vi "Engine Config Cluster to DSF Config File.vi"(8 "error in (no error)":errorcluster, 10 "dsf configuration file path":path, 11 "framework configuration":T1) -> (0 "error out":errorcluster)   [LabVIEW 2017, in "DSF Core.lvlib" / "Configuration Session.lvclass"]
uses:
  Configuration/Configuration Session.lvclass
  Configuration/Public/Controls/DSF Engine Framework Configuration.ctl
  Configuration/Public/Controls/DSF Engine Plugin Configuration.ctl
  Configuration/Public/Controls/DSF Timing Info.ctl
  Configuration/Public/Controls/DSF Engine Transfer Group Configuration.ctl
  Configuration/Public/Controls/DSF Direction.ctl
  Configuration/Public/Controls/DSF Engine Transfer Configuration.ctl
  Configuration/Public/Controls/DSF Byte Order.ctl
  Configuration/Public/Controls/DSF Engine Channel Configuration.ctl
  Configuration/Public/Controls/DSF Data Type.ctl
  Configuration/Public/Controls/DSF Settings Info.ctl
  Configuration/Public/Controls/DSF Plugin Info.ctl
  Configuration/Public/Controls/DSF Group Info.ctl
  Configuration/Public/Controls/DSF Transfer Info.ctl
  Configuration/Public/Controls/DSF Channel Info.ctl
  Configuration/Public/Write Item/Write Channel.vi
  Configuration/Public/Write Item/Write Transfer.vi
  Configuration/Public/Write Item/Write Group.vi
  Configuration/Public/Write Item/Write Plugin.vi
  DSF Core.lvlib
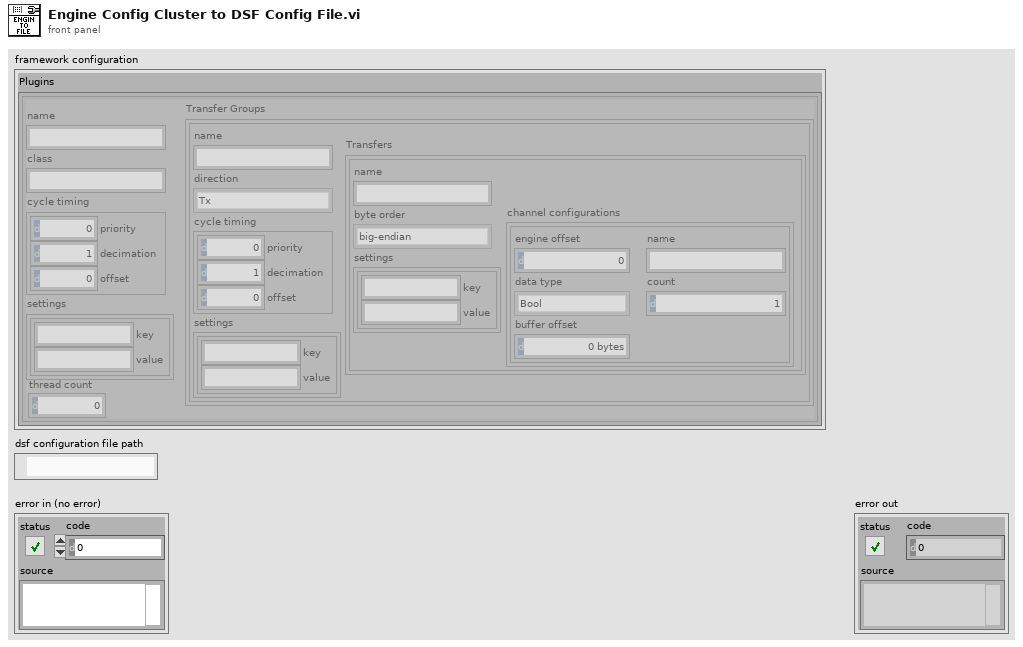
[diagram p1: front panel]
types:
  T1 = typedef "DSF Core.lvlib/DSF Engine Framework Configuration.ctl" = cluster{"Plugins":T2[]}
  T2 = typedef "DSF Core.lvlib/DSF Engine Plugin Configuration.ctl" = cluster{"name":string, "class":string, "cycle timing":T3, "Transfer Groups":T4[], "settings":T10, "thread count":i32}
  T3 = typedef "DSF Core.lvlib/DSF Timing Info.ctl" = cluster{"priority":u64, "decimation":u64, "offset":u64}
  T4 = typedef "DSF Core.lvlib/DSF Engine Transfer Group Configuration.ctl" = cluster{"name":string, "direction":T5, "cycle timing":T3, "Transfers":T6[], "settings":T10}
  T5 = typedef "DSF Core.lvlib/DSF Direction.ctl" = enum8{"Tx", "Rx"}
  T6 = typedef "DSF Core.lvlib/DSF Engine Transfer Configuration.ctl" = cluster{"name":string, "byte order":T7, "channel configurations":T8[], "settings":T10}
  T7 = typedef "DSF Core.lvlib/DSF Byte Order.ctl" = enum8{"big-endian", "little-endian"}
  T8 = typedef "DSF Core.lvlib/DSF Engine Channel Configuration.ctl" = cluster{"engine offset":u64, "name":string, "data type":T9, "count":u64, "buffer offset":u64}
  T9 = typedef "DSF Core.lvlib/DSF Data Type.ctl" = enum8{"Bool", "SGL", "DBL", "I8", "I16", "I32", "I64", "U8", "U16", "U32", "U64"}
  T10 = typedef "DSF Core.lvlib/DSF Settings Info.ctl" = cluster{"key":string, "value":string}[]
  T11 = typedef "DSF Core.lvlib/DSF Plugin Info.ctl" = cluster{"type":string, "timing":T3, "group ids":string[], "settings id":string, "thread count":i32}
  T12 = typedef "DSF Core.lvlib/DSF Group Info.ctl" = cluster{"direction":T5, "timing":T3, "transfer ids":string[], "settings id":string}
  T13 = typedef "DSF Core.lvlib/DSF Transfer Info.ctl" = cluster{"byte order":T7, "channel ids":string[], "settings id":string}
  T14 = typedef "DSF Core.lvlib/DSF Channel Info.ctl" = cluster{"count":u64, "buffer offset":u64, "data type":T9, "settings id":string}
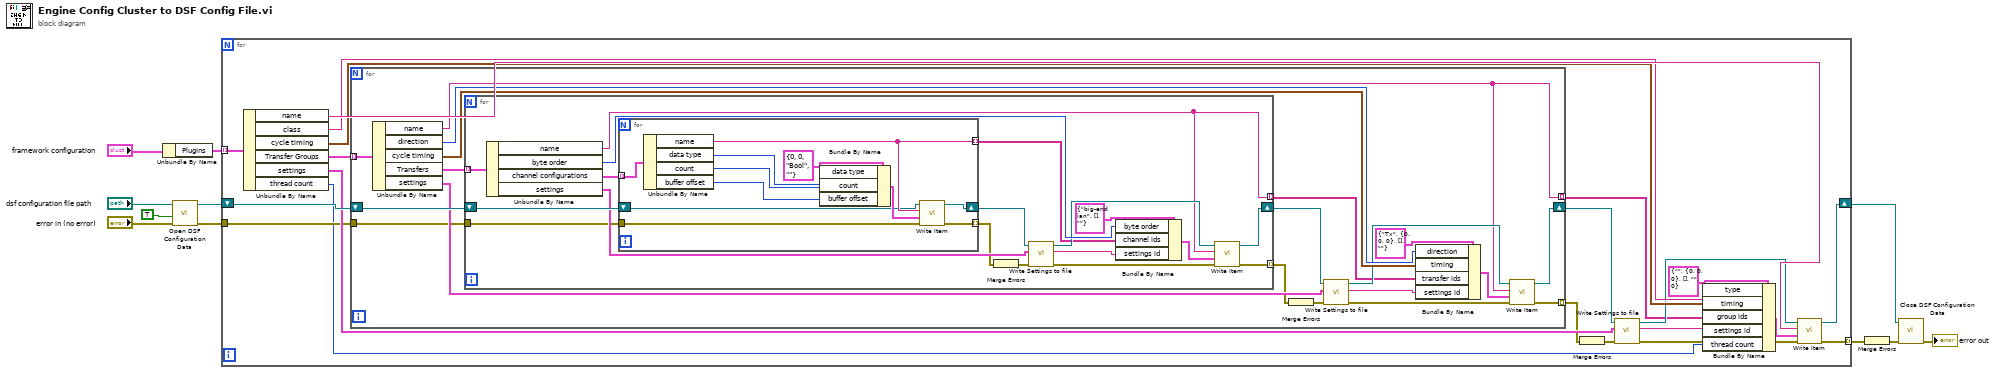
[diagram p0: block diagram]
diagram:
  n1 = Unbundle By Name("framework configuration") -> ("Plugins"=w7:T2[])
  n2 = call "Open DSF Configuration Data.vi"("error in (no error)"="error in (no error)", "replace if found? (F)"=TRUE, "dsf configuration file path"="dsf configuration file path") -> ("error out"=w4:errorcluster, "Configuration Session"=w6:refnum<class "Configuration Session.lvclass">)  [unwired: 4 in, 3 out]
  n3 = for {
    tunnel: w7 -> [w31] mode=indexing
    shift-right: [w23] -> w5
    shift-left: w6 -> [w24]
    tunnel: w4 -> [w17]
    tunnel: [w14] -> w3 mode=indexing
    n4 = Unbundle By Name(w31) -> ("name"=w30:string, "class"=w27:string, "cycle timing"=w26:T3, "Transfer Groups"=w25:T4[], "settings"=w21:T10, "thread count"=w12:i32)
    n5 = for {
      tunnel: w25 -> [w50] mode=indexing
      shift-right: [w42] -> w19
      shift-left: w24 -> [w44]
      tunnel: [w37] -> w18 mode=indexing
      tunnel: w17 -> [w36]
      tunnel: [w35] -> w16 mode=indexing
      n6 = Unbundle By Name(w50) -> ("name"=w37:string, "direction"=w47:T5, "cycle timing"=w46:T3, "Transfers"=w45:T6[], "settings"=w40:T10)
      n7 = for {
        tunnel: w45 -> [w68] mode=indexing
        shift-right: [w61] -> w43
        shift-left: w44 -> [w63]
        tunnel: [w56] -> w38 mode=indexing
        tunnel: w36 -> [w55]
        tunnel: [w52] -> w34 mode=indexing
        n8 = Unbundle By Name(w68) -> ("name"=w56:string, "byte order"=w66:T7, "channel configurations"=w64:T8[], "settings"=w59:T10)
        n9 = for {
          tunnel: w64 -> [w79] mode=indexing
          shift-right: [w73] -> w62
          shift-left: w63 -> [w69]
          tunnel: [w72] -> w57 mode=indexing
          tunnel: w55 -> [w70]
          tunnel: [w71] -> w54 mode=indexing
          n10 = Unbundle By Name(w79) -> ("name"=w72:string, "data type"=w77:T9, "count"=w76:u64, "buffer offset"=w75:u64)
          n11 = Bundle By Name(cluster=T14 {"count"=0, "buffer offset"=0, "data type"=enum."Bool", "settings id"=""} ("values"), "data type"=w77, "count"=w76, "buffer offset"=w75) -> (w74:T14)
          n12 = call-poly "Write Item.vi"("error in (no error)"=w70, "channel values"=w74, "id"=w72, "Configuration Session in"=w69) -> ("error out"=w71:errorcluster, "Configuration Session out"=w73:refnum<class "Configuration Session.lvclass">)  [unwired: 5 in, 1 out]
        }
        n13 = Merge Errors(w54) -> (w51:errorcluster)
        n14 = call "Write Settings to file.vi"("error in (no error)"=w51, "settings"=w59, "Configuration Session in"=w62) -> ("error out"=w53:errorcluster, "settings id"=w58:string, "Configuration Session out"=w60:refnum<class "Configuration Session.lvclass">)  [unwired: 6 in]
        n15 = Bundle By Name(cluster=T13 {"byte order"=enum."big-endian", "channel ids"=[], "settings id"=""} ("values"), "byte order"=w66, "channel ids"=w57, "settings id"=w58) -> (w65:T13)
        n16 = call-poly "Write Item.vi"("error in (no error)"=w53, "transfer values"=w65, "id"=w56, "Configuration Session in"=w60) -> ("error out"=w52:errorcluster, "Configuration Session out"=w61:refnum<class "Configuration Session.lvclass">)  [unwired: 5 in, 1 out]
      }
      n17 = Merge Errors(w34) -> (w32:errorcluster)
      n18 = call "Write Settings to file.vi"("error in (no error)"=w32, "settings"=w40, "Configuration Session in"=w43) -> ("error out"=w33:errorcluster, "settings id"=w39:string, "Configuration Session out"=w41:refnum<class "Configuration Session.lvclass">)  [unwired: 6 in]
      n19 = Bundle By Name(cluster=T12 {"direction"=enum."Tx", "timing"={"priority"=0, "decimation"=0, "offset"=0}, "transfer ids"=[], "settings id"=""} ("group values"), "direction"=w47, "timing"=w46, "transfer ids"=w38, "settings id"=w39) -> (w48:T12)
      n20 = call-poly "Write Item.vi"("error in (no error)"=w33, "group values"=w48, "id"=w37, "Configuration Session in"=w41) -> ("error out"=w35:errorcluster, "Configuration Session out"=w42:refnum<class "Configuration Session.lvclass">)  [unwired: 5 in, 1 out]
    }
    n21 = Merge Errors(w16) -> (w13:errorcluster)
    n22 = call "Write Settings to file.vi"("error in (no error)"=w13, "settings"=w21, "Configuration Session in"=w19) -> ("error out"=w15:errorcluster, "settings id"=w22:string, "Configuration Session out"=w20:refnum<class "Configuration Session.lvclass">)  [unwired: 6 in]
    n23 = Bundle By Name(cluster=T11 {"type"="", "timing"={"priority"=0, "decimation"=0, "offset"=0}, "group ids"=[], "settings id"="", "thread count"=0} ("plugin values"), "type"=w27, "timing"=w26, "group ids"=w18, "settings id"=w22, "thread count"=w12) -> (w28:T11)
    n24 = call-poly "Write Item.vi"("error in (no error)"=w15, "plugin values"=w28, "id"=w30, "Configuration Session in"=w20) -> ("error out"=w14:errorcluster, "Configuration Session out"=w23:refnum<class "Configuration Session.lvclass">)  [unwired: 5 in, 1 out]
  }
  n25 = Merge Errors(w3) -> (w1:errorcluster)
  n26 = call "Close DSF Configuration Data.vi"("error in (no error)"=w1, "Configuration Session"=w5) -> ("error out"=→"error out":errorcluster)  [unwired: 8 in, 1 out]
